vi "SR201_get_state.vi"(7 "command":string="0\n", 8 "error in":errorcluster, 11 "conn_id_in":refnum<k5>) -> (0 "error out":errorcluster, 1 "ch2":bool, 2 "ch1":bool, 3 "conn_id_out":refnum<k5>, 4 "status":bool, 5 "string":string)   [LabVIEW 2019]
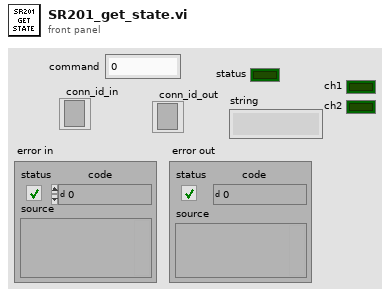
[diagram p1: front panel]
types:
  T1 = enum16{"Standard", "Buffered", "CRLF", "Immediate"}
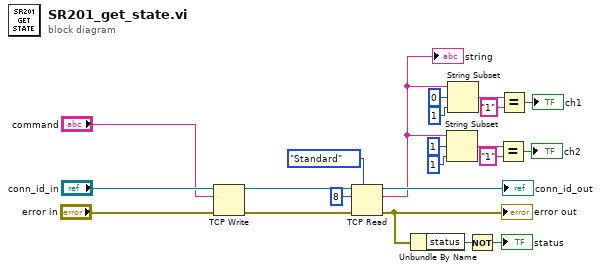
[diagram p0: block diagram]
diagram:
  n1 = TCP Write(connection ID="conn_id_in", data in="command", error in (no error)="error in") -> (connection ID out=w20:refnum<k5>, error out=w21:errorcluster)  [unwired: 1 in, 1 out]
  n2 = TCP Read(connection ID=w20, bytes to read=8, error in (no error)=w21, 7:T1."Standard" ("mode (standard)")) -> (connection ID out=→"conn_id_out":refnum<k5>, data out=w1:string, error out=w14:errorcluster)  [unwired: 1 in]
  "error out" <- w14
  "string" <- w1
  n3 = Unbundle By Name(w14) -> ("status"=w13:bool)
  n4 = String Subset(string=w1, offset (0)=1, length (rest)=1 ("length (rest)")) -> (substring=w4:string)
  n5 = String Subset(string=w1, offset (0)=0, length (rest)=1 ("length (rest)")) -> (substring=w9:string)
  n6 = Not(x=w13) -> (.not. x?=→"status":bool)
  n7 = Equal?(x=w4, y="1") -> (x = y?=→"ch2":bool)
  n8 = Equal?(x=w9, y="1") -> (x = y?=→"ch1":bool)
